vi "PIM Init MeasStatusBar.vi"(1 "Meas Status":refnum<vi>, 11 "error in (no error)":errorcluster, 12 "Meas Params":T1={"IM Order"=0, "Direction"=0, "Averaging"=1, "ALC ON?"=TRUE, "Peak Hold?"=TRUE, "Peak last N"=0, "Ref Level dBm"=0.0, "Ref Units"=enum."dBm", "Num Samples"=0, "Sample units"=enum."Sample(s)", "Update Rate (s)"=0.0, "DUT PORT"=enum."Port 1", "Percent (%)"=100} {"Averaging" items=["None", "Minimum", "Normal", "High", "Maximum"]; "Direction" items=["Reverse", "Forward", "Auxiliary"]; "IM Order" items=["3rd", "5th", "7th", "9th", "11th", "13th", "15th", "17th", "19th", "21st", "23rd", "25th", "27th", "29th", "31st", "33rd"]}) -> (15 "error out":errorcluster)   [LabVIEW 2011]
uses:
  TypeDefs/PIM Meas Status Bar.ctl
  TypeDefs/PIM Measurement Parameters.ctl
  BPIMCore/HW IO/IMOrder.ctl
  BPIMCore/HW IO/MeasMode.ctl
  BPIMCore/HW IO/HW Averaging.ctl
  TypeDefs/PIM Meas Units.ctl
  BPIMCore/HW IO/DUTport.ctl
panel:
  out "Meas Status 3":T7
  out "Meas Status 2":T7
  out "Meas Status":T7
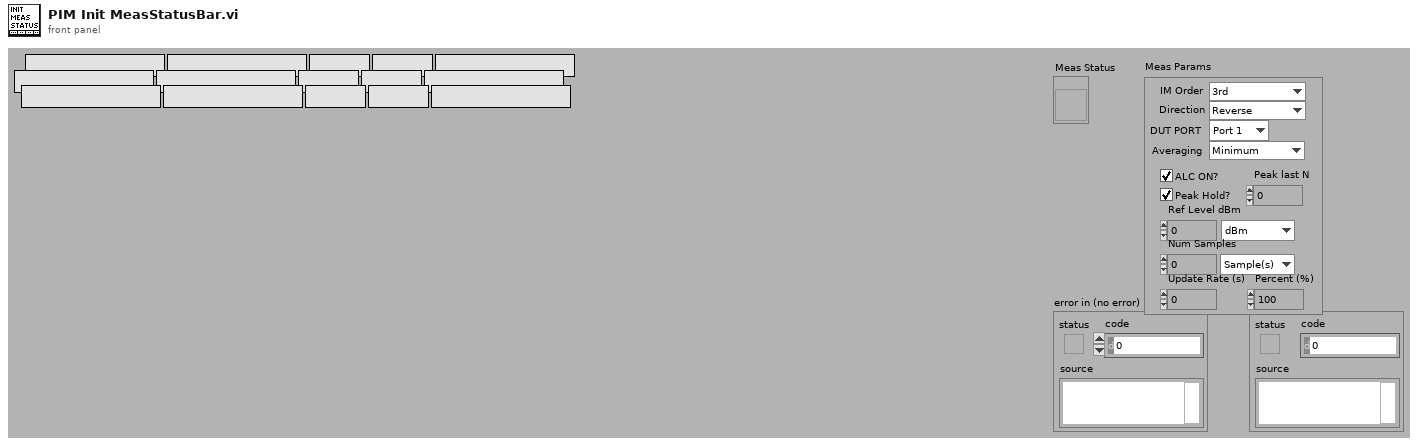
[diagram p1: front panel]
types:
  T1 = typedef "PIM Measurement Parameters.ctl" = cluster{"IM Order":T2, "Direction":T3, "Averaging":T4, "ALC ON?":bool, "Peak Hold?":bool, "Peak last N":u32, "Ref Level dBm":dbl, "Ref Units":enum16{"dBm", "dBc"}, "Num Samples":u32, "Sample units":T5, "Update Rate (s)":dbl, "DUT PORT":T6, "Percent (%)":u8}
  T2 = typedef "IMOrder.ctl" = u8
  T3 = typedef "MeasMode.ctl" = u16
  T4 = typedef "HW Averaging.ctl" = u16
  T5 = typedef "PIM Meas Units.ctl" = enum16{"Sample(s)", "Second(s)", "Sweep(s)"}
  T6 = typedef "DUTport.ctl" = enum16{"Port 1", "Port 2"}
  T7 = typedef "PIM Meas Status Bar.ctl" = cluster{"Date":string, "Averaging":string, "ALC":string, "IM Order":string, "Measure Direction":string}
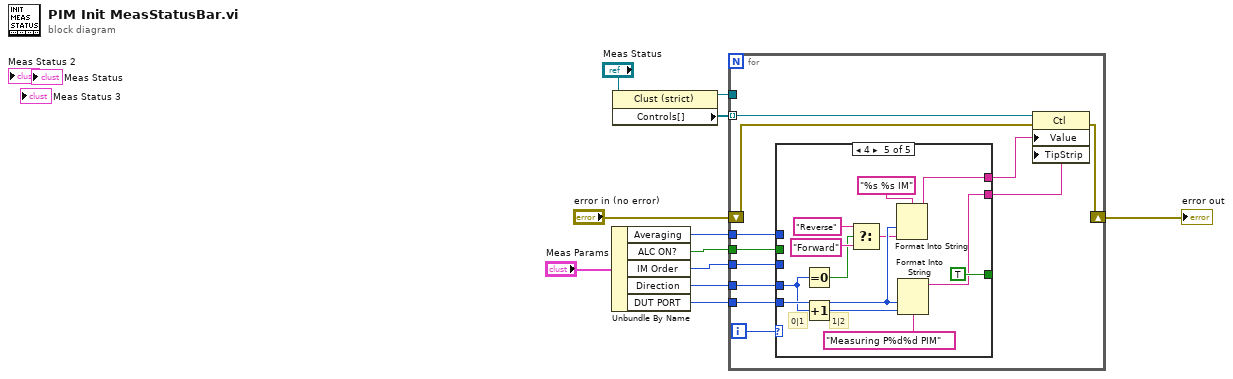
[diagram p0: block diagram]
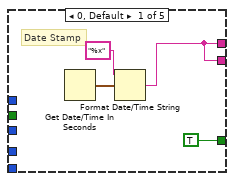
[diagram p2: hidden frame]
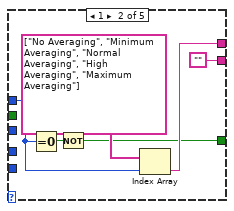
[diagram p3: hidden frame]
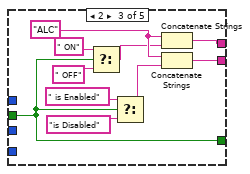
[diagram p4: hidden frame]
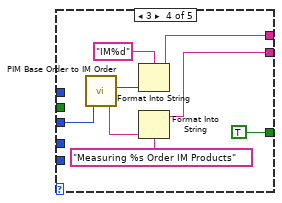
[diagram p5: hidden frame]
diagram:
  n1 = Unbundle By Name("Meas Params") -> ("Averaging"=w5:T4, "ALC ON?"=w4:bool, "IM Order"=w3:T2, "Direction"=w2:T3, "DUT PORT"=w1:T6)
  n2 = property class="Clust (strict)"(reference="Meas Status") -> (reference out=w8:refnum<vi>, "Controls[]"=w7:refnum<vi>[])  [unwired: 1 in, 1 out]
  n3 = for {
    shift-right: [w15] -> w11
    shift-left: "error in (no error)" -> [w14]
    tunnel: w5 -> [w22]
    tunnel: w4 -> [w21]
    tunnel: w3 -> [w20]
    tunnel: w2 -> [w19]
    tunnel: w8 -> [_]
    tunnel: w7 -> [w18] mode=indexing
    tunnel: w1 -> [w12]
    i -> [w13]
    n4 = case shown="4" w13 {
      tunnel: [w23 w31 w37 w44 w52] -> w17
      tunnel: [w23 "" w39 w47 w51] -> w16
      tunnel: w22 -> [_ w30 _ _ _]
      tunnel: [TRUE ("ALC ON?") w28 w34 TRUE ("ALC ON?") TRUE ("ALC ON?")] -> _
      tunnel: w21 -> [_ _ w34 _ _]
      tunnel: w20 -> [_ _ _ w50 _]
      tunnel: w19 -> [_ _ _ _ w54]
      tunnel: w12 -> [_ _ _ _ w58]
      frame 0, Default {
        # "Date Stamp"
        n5 = Get Date/Time In Seconds() -> (seconds since 1Jan1904=w25:timestamp)
        n6 = Format Date/Time String(time format string (%c)="%x", seconds (now)=w25) -> (date/time string=w23:string)  [unwired: 1 out]
      }
      frame 1 {
        n7 = Equal To 0?(x=w30) -> (x = 0?=w29:bool)
        n8 = Not(x=w29) -> (.not. x?=w28:bool)
        n9 = Index Array(array=string[] ["No Averaging", "Minimum Averaging", "Normal Averaging", "High Averaging", "Maximum Averaging"], index=w30) -> (element=w31:string)
      }
      frame 2 {
        w38 = "ALC"
        n10 = Select(t=" ON", s=w34, f=" OFF") -> (s? t:f=w33:string)
        n11 = Select(t=" is Enabled", s=w34, f="is Disabled") -> (s? t:f=w40:string)
        n12 = Concatenate Strings(w38, w33) -> (w37:string)
        n13 = Concatenate Strings(w38, w40) -> (w39:string)
      }
      frame 3 {
        n14 = call "PIM Base Order to IM Order.vi"("Base Order (0)"=w50) -> ("IM Order"=w45:u8, "IM Order String"=w48:string)  [unwired: 4 out]
        n15 = Format Into String(format string="IM%d", w45) -> (resulting string=w44:string)  [unwired: 2 in, 1 out]
        n16 = Format Into String(format string="Measuring %s Order IM Products", w48) -> (resulting string=w47:string)  [unwired: 2 in, 1 out]
      }
      frame 4 {
        # "1|2"
        # "0|1"
        n17 = Equal To 0?(x=w54) -> (x = 0?=w53:bool)
        n18 = Increment(x=w54) -> (x+1=w59:T3)
        n19 = Select(t="Reverse" ("format string"), s=w53, f="Forward" ("format string")) -> (s? t:f=w57:string)
        n20 = Format Into String(format string="%s %s IM", w58, w57) -> (resulting string=w52:string)  [unwired: 2 in, 1 out]
        n21 = Format Into String(format string="Measuring P%d%d PIM", w58, w59) -> (resulting string=w51:string)  [unwired: 2 in, 1 out]
      }
    }
    n22 = property class="Ctl"(reference=w18, error in=w14, "Value"=w17, "TipStrip"=w16) -> (error out=w15:errorcluster)  [unwired: 1 out]
  }
  "error out" <- w11
